vi "Configure Sequence (Exponential).vi"(0 "VISA resource name":refnum<visa-resource-name>, 1 "Channel Name (1)":string="1", 3 "Exponential Sequence Time Constant (1.0)":dbl=1.0 format="%^.3e", 4 "Waveform Type (1: Voltage)":i32(ring)=1 items=["Voltage"=1, "Current"=0], 5 "error in (no error)":errorcluster {"code" format="%.0x"}, 6 "Exponential Sequence Start Time (0.0 s)":dbl format="%^.3e", 7 "Exponential Sequence Total Time (1.0 s)":dbl=1.0 format="%^.3e", 8 "Exponential Sequence Start Level (0.0)":dbl format="%^.3e", 9 "Exponential Sequence End Level (0.0)":dbl format="%^.3e", 12 "Sequence Step Number (0)":i32) -> (14 "VISA resource name out":refnum<visa-resource-name>, 19 "error out":errorcluster {"code" format="%.0x"})   [LabVIEW 2010, in "Agilent N6700 Series.lvlib"]
doc: "This VI configures the exponential sequence.\n\n<b>Note:</b>\n\nSequence capability is only available on the N6705B DC Power Analyzer."
uses:
  Agilent N6700 Series.lvlib
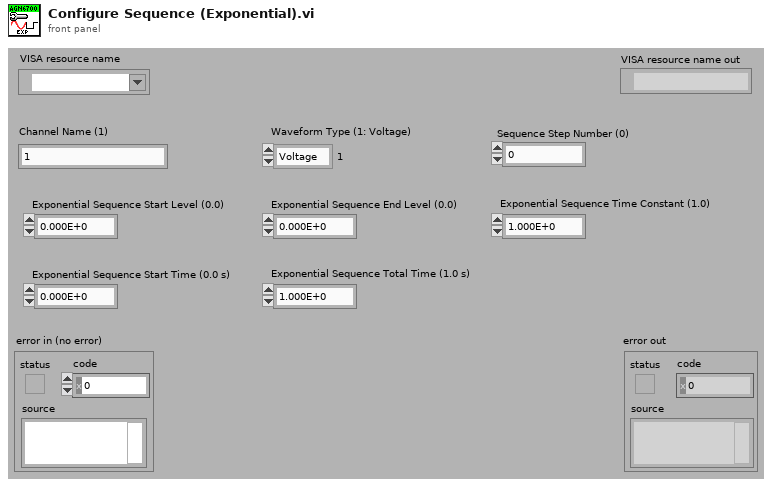
[diagram p1: front panel]
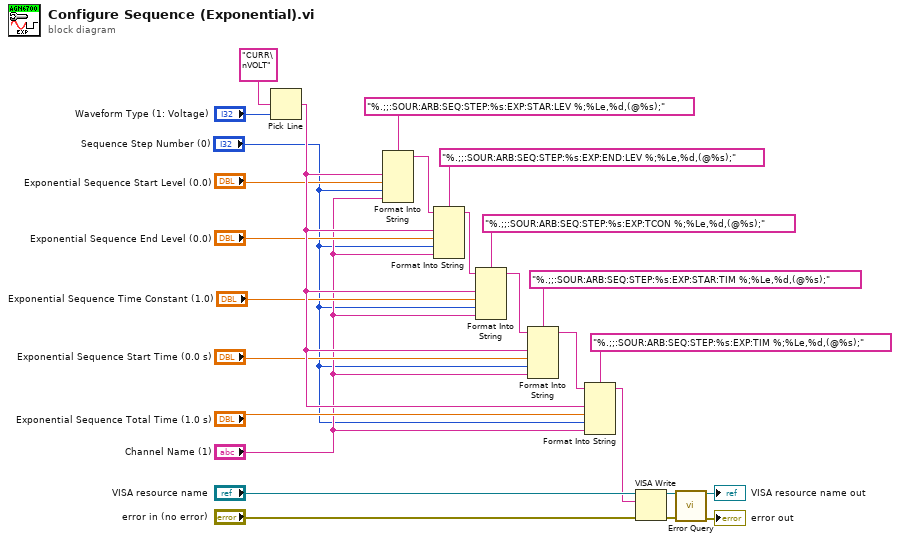
[diagram p0: block diagram]
diagram:
  n1 = Pick Line(multi-line string="CURR\nVOLT", line index="Waveform Type (1: Voltage)") -> (output string=w15:string)  [unwired: 1 in]
  n2 = Format Into String(format string="%.;;:SOUR:ARB:SEQ:STEP:%s:EXP:STAR:LEV %;%Le,%d,(@%s);", w15, "Exponential Sequence Start Level (0.0)", "Sequence Step Number (0)", "Channel Name (1)") -> (resulting string=w19:string)  [unwired: 2 in, 1 out]
  n3 = Format Into String(format string="%.;;:SOUR:ARB:SEQ:STEP:%s:EXP:END:LEV %;%Le,%d,(@%s);", initial string=w19, w15, "Exponential Sequence End Level (0.0)", "Sequence Step Number (0)", "Channel Name (1)") -> (resulting string=w18:string)  [unwired: 1 in, 1 out]
  n4 = Format Into String(format string="%.;;:SOUR:ARB:SEQ:STEP:%s:EXP:TCON %;%Le,%d,(@%s);", initial string=w18, w15, "Exponential Sequence Time Constant (1.0)", "Sequence Step Number (0)", "Channel Name (1)") -> (resulting string=w17:string)  [unwired: 1 in, 1 out]
  n5 = Format Into String(format string="%.;;:SOUR:ARB:SEQ:STEP:%s:EXP:STAR:TIM %;%Le,%d,(@%s);", initial string=w17, w15, "Exponential Sequence Start Time (0.0 s)", "Sequence Step Number (0)", "Channel Name (1)") -> (resulting string=w16:string)  [unwired: 1 in, 1 out]
  n6 = Format Into String(format string="%.;;:SOUR:ARB:SEQ:STEP:%s:EXP:TIM %;%Le,%d,(@%s);", initial string=w16, w15, "Exponential Sequence Total Time (1.0 s)", "Sequence Step Number (0)", "Channel Name (1)") -> (resulting string=w14:string)  [unwired: 1 in, 1 out]
  n7 = VISA Write(VISA resource name="VISA resource name", write buffer=w14, error in (no error)="error in (no error)") -> (VISA resource name out=w23:refnum<visa-resource-name>, error out=w22:errorcluster)  [unwired: 1 out]
  n8 = call "Error Query.vi"("VISA resource name"=w23, "error in (no error)"=w22) -> ("VISA resource name out"=→"VISA resource name out":refnum<visa-resource-name>, "error out"=→"error out":errorcluster)  [unwired: 10 in, 2 out]
